vi "stopping Controller.vi"(8 "error in":errorcluster) -> ()   [LabVIEW 2020]
doc: "This VI executes continuously carrying out the current operation and responding to updates or new operations. It will often contain the timing or control code that is difficult to place directly in TeleOp. This VI generally opens all sensors and motors and isolates the rest of the robot code from knowing how the operations are carried out."
uses:
  <vilib>/Rock Robotics/WPI/Framework/Completion Status.ctl
  stopping Setpoints.ctl
  stopping Operations.ctl
  Framework/Robot Global Data.vi
  <vilib>/Rock Robotics/Network Tables/NT Write Boolean.vi
panel:
  in  "Interactive Values":T1
  out "Current\nCmd":string
  in  "Buttons":cluster{"Execute Cmd":bool, "Abort Cmd":bool}
  out "Command Timing":cluster{"Start Time (ms)":u32, "Iterations":i32}
  out "Status":T3
  # "Tip: It may be helpful to observe inputs and sensor values.\nYou may also want to display tuning or debugging controls."
  # "Interactive Command: You may fill in the settings for a command\nand schedule it with the Execute button. You can observe and abort\nany command while fine tuning the code for the controller."
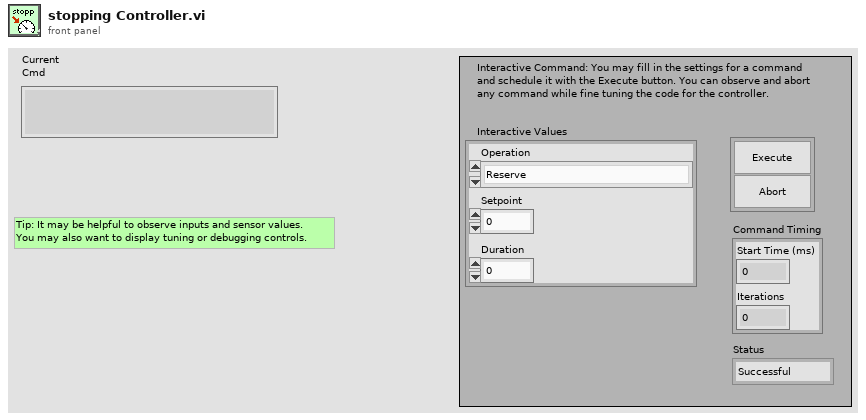
[diagram p1: front panel]
types:
  T1 = typedef "stopping Setpoints.ctl" = cluster{"Operation":T2, "Setpoint":dbl, "Duration":dbl}
  T2 = typedef "stopping Operations.ctl" = enum16{"Reserve", "Read Current", "Immediate", "stop"}
  T3 = typedef "Completion Status.ctl" = enum16{"Successful", "Aborted", "Incomplete"}
  T4 = typedef "Command Status Info.ctl" = cluster{"Name":string, "Status":T3, "notifier out":T5}
  T5 = typedef "Completion Notifier.ctl" = refnum<notifier>
  T6 = cluster{"Current Command":T1, "Command Timing":cluster{"Start Time (ms)":u32, "Iterations":i32}, "Command Arguments":cluster{"Command Info":T4, "Description":string, "Default Command":T1, "queue out":refnum<queue>, "Subsystem Name":string}}
  T7 = typedef "Color Sensor V3 DevRef.ctl" = cluster{"I2CDevRef":T8}
  T8 = typedef "WPI_I2CDevRef.ctl" = cluster{"DevStatus":errorcluster, "Device Address":u8, "Handle":i32, "I2C Bus":T9}
  T9 = typedef "i2c_bus.ctl" = enum16{"I2C On-Board", "I2C MXP", "Invalid"}
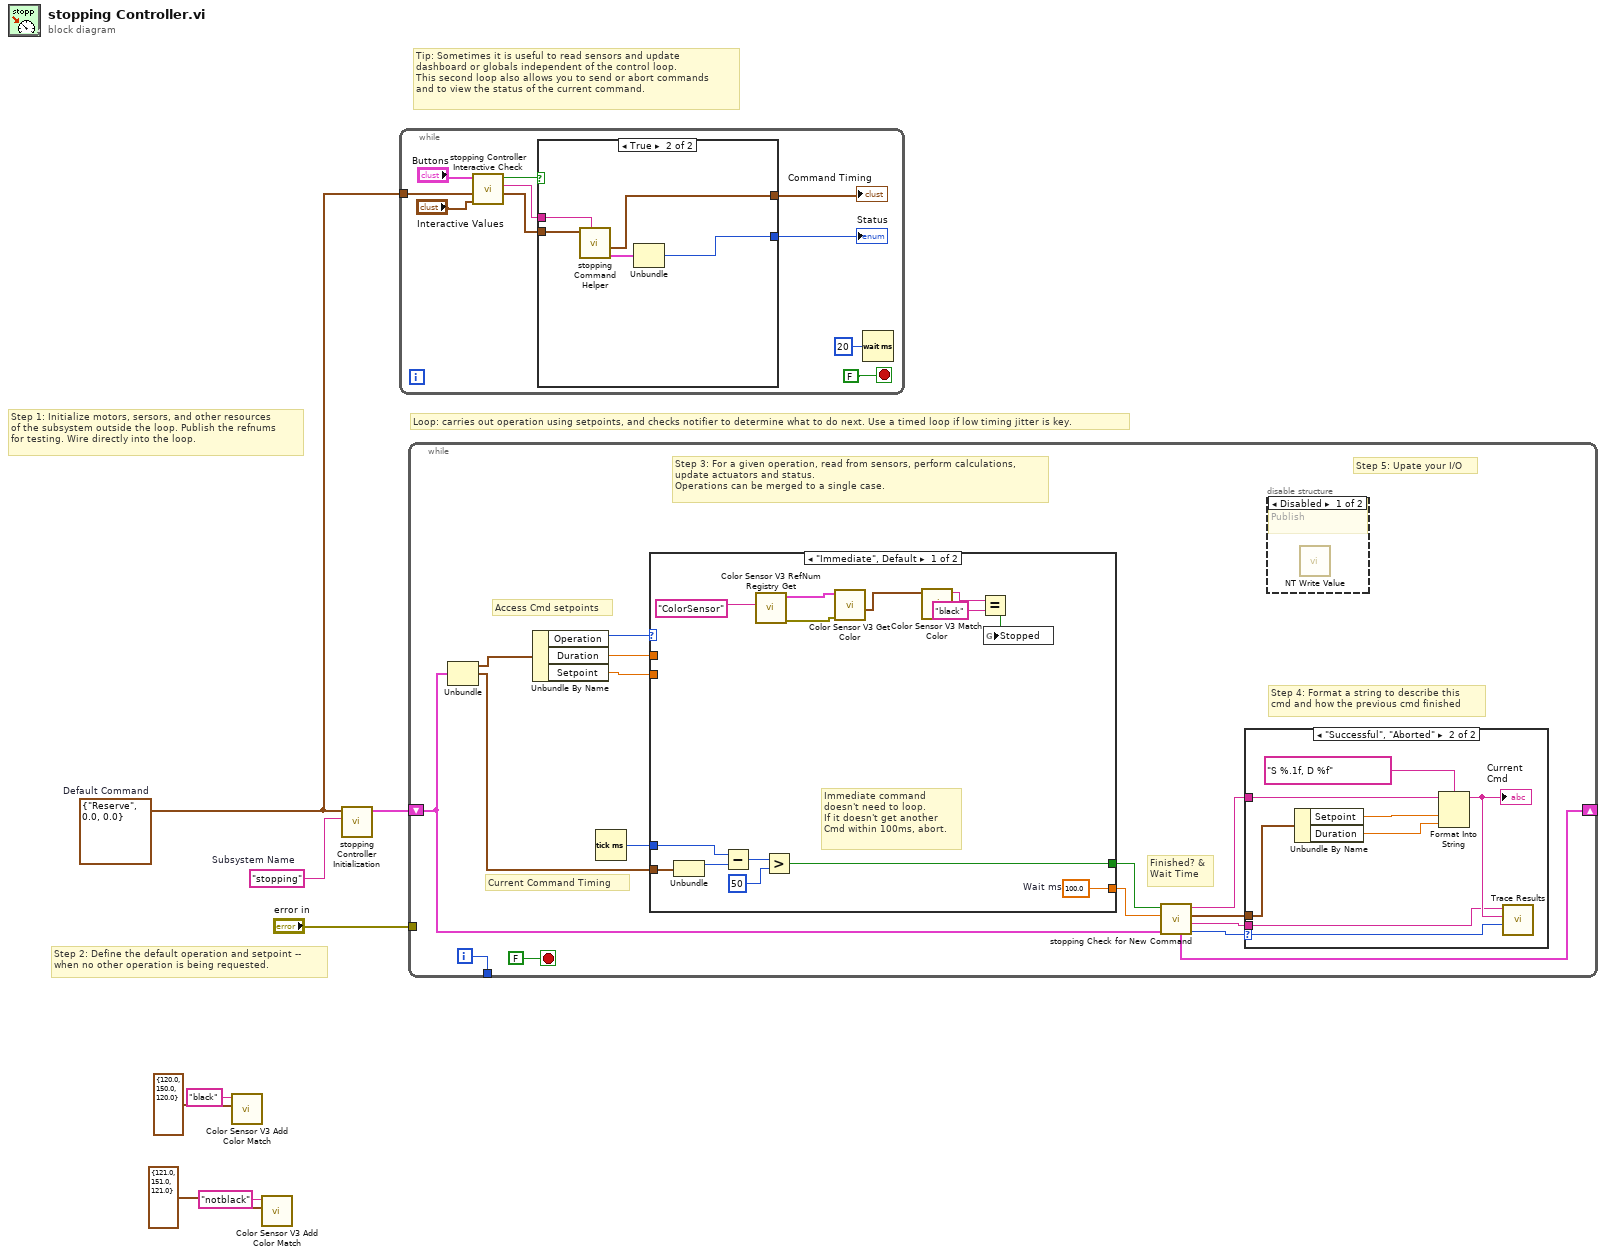
[diagram p0: block diagram]
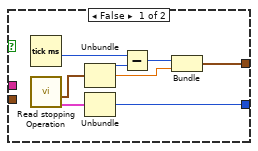
[diagram p2: hidden frame]
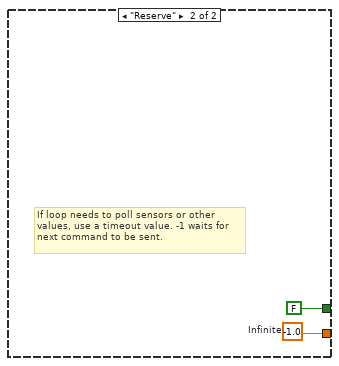
[diagram p5: hidden frame]
diagram:
  w5 = T1 {"Operation"=enum."Reserve", "Setpoint"=0.0, "Duration"=0.0}  # Default Command
  w6 = "stopping"  # Subsystem Name
  # "Tip: Sometimes it is useful to read sensors and update\ndashboard or globals independent of the control loop.\nThis second loop also allows you to send or abort commands\nand to view the status of the current command."
  # "Step 2: Define the default operation and setpoint --\nwhen no other operation is being requested."
  # "Step 1: Initialize motors, sersors, and other resources\nof the subsystem outside the loop. Publish the refnums\nfor testing. Wire directly into the loop."
  # "Loop: carries out operation using setpoints, and checks notifier to determine what to do next. Use a timed loop if low timing jitter is key."
  n1 = call <vilib>:"Color Sensor V3 Add Color Match.vi"("Color"=cluster{"R":dbl, "G":dbl, "B":dbl} {"R"=120.0, "G"=150.0, "B"=120.0}, "Name"="black") -> ()  [unwired: 10 in]
  n2 = call <vilib>:"Color Sensor V3 Add Color Match.vi"("Color"=cluster{"R":dbl, "G":dbl, "B":dbl} {"R"=121.0, "G"=151.0, "B"=121.0}, "Name"="notblack") -> ()  [unwired: 10 in]
  n3 = call "stopping Controller Initialization.vi"("Subsystem Name"=w6, "Default Command"=w5) -> ("Current Command"=w7:T6)  [unwired: 9 in]
  n4 = while {
    tunnel: w5 -> [w15]
    stop <- FALSE stop-if-true
    n5 = call "stopping Controller Interactive Check.vi"("Interactive Command in"="Interactive Values", "Default Command"=w15, "Buttons"="Buttons") -> ("Interactive Command out"=w12:T1, "Trace String"=w13:string, "Schedule"=w14:bool)  [unwired: 6 in]
    n6 = case shown="True" w14 {
      tunnel: [w26 w31] -> w11
      tunnel: w12 -> [_ w29]
      tunnel: [w22 w27] -> w10
      tunnel: w13 -> [_ w30]
      frame False {
        n7 = Tick Count (ms)() -> (millisecond timer value=w21:u32)
        n8 = call "Read stopping Operation.vi"() -> ("Command Info"=w19:T4, "SubSystem Data"=w20:T1)  [unwired: 9 in, 1 out]
        n9 = Unbundle(w20) -> ("Operation"=w25:T2, "Setpoint"=w23:dbl)  [unwired: 1 out]
        n10 = Unbundle(w19) -> ("Status"=w26:T3)  [unwired: 2 out]
        n11 = Subtract(x=w21, y=w25) -> (x-y=w24:u32)
        n12 = Bundle(w24, "Setpoint"=w23) -> (w22:cluster{u32, "Setpoint":dbl})  [unwired: 1 in]
      }
      frame True {
        n13 = call "stopping Command Helper.vi"("Description"=w30, "SubSystem Data"=w29) -> ("Command Info Out"=w28:T4, "Command Timing"=w27:cluster{"Start Time (ms)":u32, "Iterations":i32})  [unwired: 7 in, 1 out]
        n14 = Unbundle(w28) -> ("Status"=w31:T3)  [unwired: 2 out]
      }
    }
    "Status" <- w11
    "Command Timing" <- w10
    n15 = Wait (ms)(milliseconds to wait=u32 20) -> ()  [unwired: 1 out]
  }
  n16 = while {
    shift-right: [w39] -> _
    shift-left: w7 -> [w32]
    tunnel: [w46] -> _
    tunnel: "error in" -> [_]
    i -> [w46]
    stop <- FALSE stop-if-true
    # "Step 5: Upate your I/O"
    # "Step 4: Format a string to describe this\ncmd and how the previous cmd finished"
    # "Current Command Timing"
    # "Access Cmd setpoints"
    # "Finished? &\nWait Time"
    # "Step 3: For a given operation, read from sensors, perform calculations,\nupdate actuators and status.\nOperations can be merged to a single case."
    n17 = Unbundle(w32) -> ("Current Command"=w45:T1, "Command Timing"=w41:cluster{"Start Time (ms)":u32, "Iterations":i32})  [unwired: 1 out]
    n18 = Unbundle By Name(w45) -> ("Operation"=w44:T2, "Duration"=w43:dbl, "Setpoint"=w40:dbl)
    n19 = Tick Count (ms)() -> (millisecond timer value=w42:u32)
    n20 = case shown="\"Immediate\", Default" w44 {
      tunnel: [w69 w71] -> w37
      tunnel: [w63 FALSE ("ignore previous (F)")] -> w38
      tunnel: w41 -> [w65 _]
      tunnel: w43 -> [_ _]
      tunnel: w42 -> [w64 _]
      tunnel: w40 -> [_ _]
      frame "Immediate", Default {
        w69 = 100.0  # Wait ms
        # "Immediate command\ndoesn't need to loop.\nIf it doesn't get another\nCmd within 100ms, abort."
        n21 = Unbundle(w65) -> ("Start Time (ms)"=w68:u32)  [unwired: 1 out]
        n22 = Subtract(x=w64, y=w68) -> (x-y=w67:u32)
        n23 = call "Color Sensor V3 RefNum Registry Get.vi"("refnum name"="ColorSensor") -> ("error out"=w60:errorcluster, "ColorSensorDevRef"=w61:T7)  [unwired: 9 in]
        n24 = Greater?(x=w67, y=u8 50 ("Left Motor")) -> (0:w63:bool)
        n25 = call <vilib>:"Color Sensor V3 Get Color.vi"("error in (no error)"=w60, "ColorSensorDevRef"=w61) -> ("Normalized Color"=w59:cluster{"R":dbl, "G":dbl, "B":dbl})  [unwired: 6 in, 3 out]
        n26 = call <vilib>:"Color Sensor V3 Match Color.vi"("Measured Color"=w59) -> ("Matched Color Name"=w58:string)  [unwired: 8 in, 2 out]
        n27 = Equal?(x=w58, y="black") -> (x = y?=w56:bool)
        n28 = global write "Robot Global Data.vi" "Stopped"(w56) -> ()
      }
      frame "Reserve" {
        w71 = -1.0  # Infinite
        # "If loop needs to poll sensors or other\nvalues, use a timeout value. -1 waits for\nnext command to be sent."
      }
    }
    n29 = call "stopping Check for New Command.vi"("Current Command"=w32, "Wait time (ms)"=w37, "Finished?"=w38) -> ("Completion"=w33:T3, "Subsystem Name"=w34:string, "Current Command"=w35:T1, "Initial Trace String"=w36:string, "NextCommand"=w39:T6)  [unwired: 4 in]
    n30 = case shown="\"Successful\", \"Aborted\"" w33 {
      selector: w33 -> [_ w55]
      tunnel: w36 -> [_ w51]
      tunnel: w35 -> [_ w52]
      tunnel: w34 -> [_ w48]
      frame "Incomplete", Default {
        # "Continuing current command"
      }
      frame "Successful", "Aborted" {
        # "Report and setup for next command"
        n31 = Unbundle By Name(w52) -> ("Setpoint"=w54:dbl, "Duration"=w49:dbl)
        n32 = Format Into String(format string="S %.1f, D %f", initial string=w51, w54, w49) -> (resulting string=w50:string)  [unwired: 1 in, 1 out]
        "Current\nCmd" <- w50
        n33 = call <vilib>:"Trace Results.vi"("Status of previous command"=w55, "Description"=w50, "Subsystem"=w48) -> ()  [unwired: 9 in]
      }
    }
    n34 = disable-structure shown="Disabled" {
      frame Disabled {
        # "Publish"
        n35 = call-poly <vilib>:"NT Write Value.vi"() -> ()  [unwired: 11 in, 1 out]
      }
      frame Enabled {
      }
    }
  }
